vi "New WebSocket Client.vi"(7 "WebSocket Client in":refnum<class "WebSocket Client.lvclass">, 8 "error in (no error)":errorcluster, 11 "Port":u16) -> (0 "error out":errorcluster, 3 "WebSocket Client out":refnum<class "WebSocket Client.lvclass">)   [LabVIEW 2017, in "WebSocket Client.lvlib" / "WebSocket Client.lvclass"]
uses:
  WebSocket Client.lvclass
  WebSocket Client.lvclass/WebSocket Client.ctl
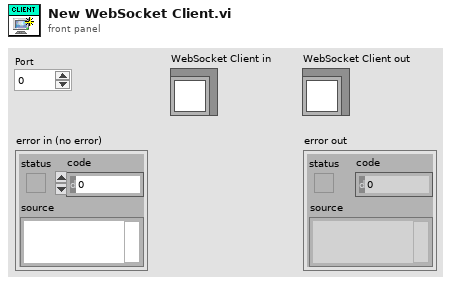
[diagram p1: front panel]
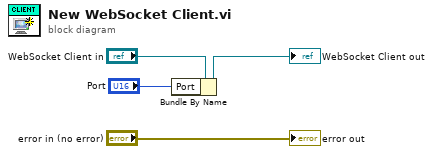
[diagram p0: block diagram]
diagram:
  n1 = Bundle By Name(cluster="WebSocket Client in", "Port"="Port") -> (→"WebSocket Client out":refnum<class "WebSocket Client.lvclass">)
  "error out" <- "error in (no error)"
